vi "Read PythonVersion.vi"(8 "error in (no error)":errorcluster, 11 "PythonSession in":refnum<class "PythonSession.lvclass">) -> (0 "error out":errorcluster, 2 "PythonVersion":string, 3 "PythonSession out":refnum<class "PythonSession.lvclass">)   [LabVIEW 2022 SP3, in "PythonWrapper.lvlib" / "PythonSession.lvclass"]
uses:
  PythonSession.lvclass
  PythonSession.lvclass/PythonSession.ctl
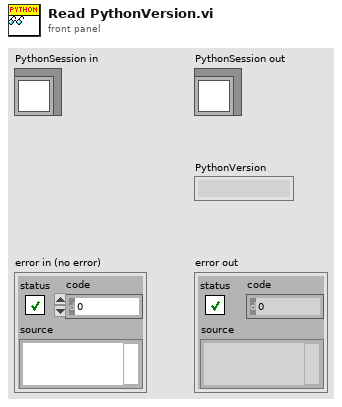
[diagram p1: front panel]
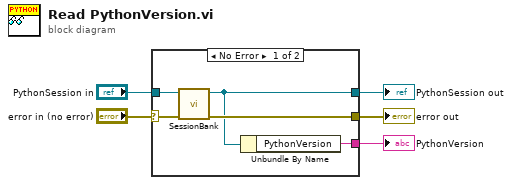
[diagram p0: block diagram]
diagram:
  n1 = case shown="No Error" "error in (no error)" {
    selector: "error in (no error)" -> [w10 w11]
    tunnel: [w8 w11] -> w2
    tunnel: [w6 w12] -> w3
    tunnel: "PythonSession in" -> [w7 w12]
    tunnel: [w9 _] -> w1
    frame No Error {
      n2 = call "SessionBank.vi"("error in (no error)"=w10, "PythonSession in"=w7) -> ("error out"=w8:errorcluster, "PythonSession out"=w6:refnum<class "PythonSession.lvclass">)  [unwired: 8 in]
      n3 = Unbundle By Name(w6) -> ("PythonVersion"=w9:string)
    }
    frame Error {
    }
  }
  "error out" <- w2
  "PythonSession out" <- w3
  "PythonVersion" <- w1
